vi "DrawLine.vi"(3 "Params":cluster{"Line width":sgl, "Line Color":u32}={"Line width"=0.03, "Line Color"=10813344}, 4 "Axes2":T1=[[1.0, 0.0, 0.0, 0.0], [0.0, 1.0, 0.0, 0.0], [0.0, 0.0, 1.0, 0.0], [0.0, 0.0, 0.0, 1.0]], 5 "Axes1":T1=[[1.0, 0.0, 0.0, 0.0], [0.0, 1.0, 0.0, 0.0], [0.0, 0.0, 1.0, 0.0], [0.0, 0.0, 0.0, 1.0]], 6 "Stage in":refnum<vi>) -> (0 "error out":errorcluster, 2 "Stage out":refnum<vi>)   [LabVIEW 2024]
uses:
  <vilib>/Analysis/Matrix/Datatypes/RealMatrix.ctl
  <vilib>/picture/3D Picture Control/NI_3D Picture Control.lvlib
  <vilib>/Analysis/Matrix/NI_Matrix.lvlib
panel:
  in  "Name":string="Undec"
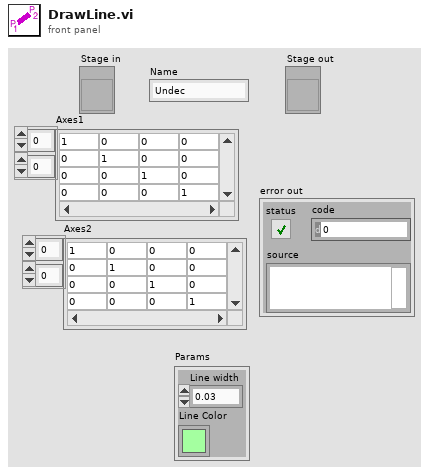
[diagram p1: front panel]
types:
  T1 = typedef "NI_Matrix.lvlib/RealMatrix.ctl" = dbl[][]
  T2 = cluster{"Axes1[0]":dbl, "Axes1[1]":dbl, "Axes1[2]":dbl}
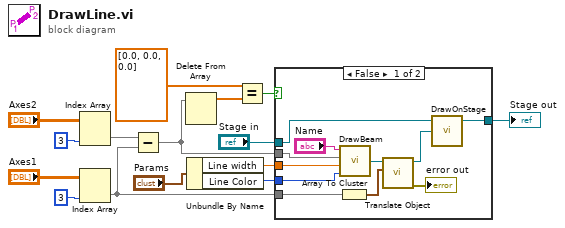
[diagram p0: block diagram]
diagram:
  n1 = Index Array(array="Axes2", index (col)=3 ("length")) -> (element=w9:dbl[])  [unwired: 1 in]
  n2 = Index Array(array="Axes1", index (col)=3 ("length")) -> (element=w6:dbl[])  [unwired: 1 in]
  n3 = Subtract ("Subtract.vi")(x=w9, y=w6) -> (x-y=w2:dbl[])
  n4 = Delete From Array(array=w2) -> (array with subset deleted=w1:dbl[])  [unwired: 2 in, 1 out]
  n5 = Unbundle By Name("Params") -> ("Line width"=w3:sgl, "Line Color"=w4:u32)
  n6 = Equal?(x=dbl[] [0.0, 0.0, 0.0] ("subarray"), y=w1) -> (x = y?=w13:bool)
  n7 = case shown="False" w13 {
    tunnel: w4 -> [w24 _]
    tunnel: w2 -> [w23 _]
    tunnel: w6 -> [w21 _]
    tunnel: [w20 w27] -> w15
    tunnel: "Stage in" -> [w19 w27]
    tunnel: w3 -> [w16 _]
    frame False {
      n8 = Array To Cluster(array=w21) -> (cluster=w25:T2)
      n9 = call <userlib>:"DrawBeam.vi"("Color"=w24, "Beam radius"=w16, "Point"=w23, "Name"="Name") -> ("Beam"=w22:refnum<vi>)  [unwired: 2 in]
      n10 = call <vilib>:"Translate Object.vi"("Translation"=w25, "Scene.Object In"=w22) -> ("error out"=→"error out":errorcluster, "Scene.Object Out"=w18:refnum<vi>)  [unwired: 8 in]
      n11 = call <userlib>:"DrawOnStage.vi"("object in"=w18, "Stage in"=w19) -> ("Stage out"=w20:refnum<vi>)  [unwired: 1 in, 2 out]
    }
    frame True {
    }
  }
  "Stage out" <- w15
